vi "Find Closest Index.vi"(10 "Time":dbl, 11 "Array":dbl[][](array[numeric])) -> (3 "Index":i32)   [LabVIEW 2015]
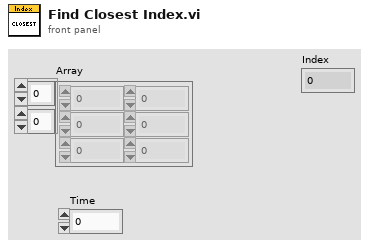
[diagram p1: front panel]
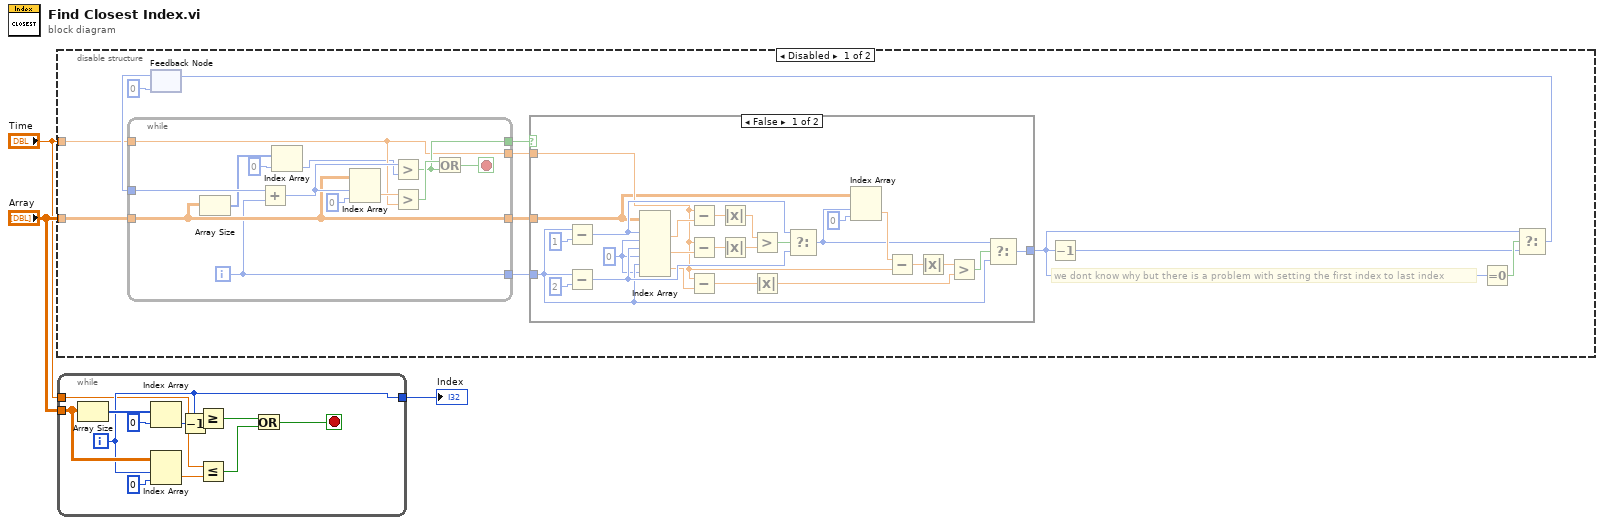
[diagram p0: block diagram]
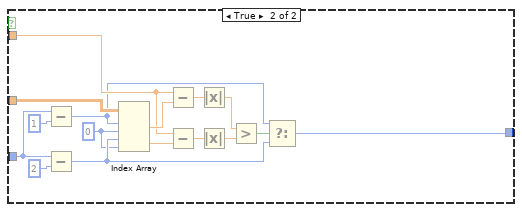
[diagram p2: hidden frame]
diagram:
  n1 = disable-structure shown="Disabled" {
    disable-tunnel: "Array" -> [w5 _]
    disable-tunnel: "Time" -> [w4 _]
    frame Disabled {
      # "we dont know why but there is a problem with setting the first index to last index"
      n2 = feedback #1(0) -> (w15:i32)
      n3 = while {
        tunnel: w5 -> [w63]
        tunnel: w15 -> [w69]
        tunnel: w4 -> [w61]
        tunnel: [w64] -> w14
        tunnel: [w63] -> w13
        tunnel: [w62] -> w12
        tunnel: [w61] -> w11
        i -> [w62]
        stop <- w65 stop-if-true
        n4 = Array Size(array=w63) -> (size(s)=w59:i32[])
        n5 = Add(x=w69, y=w62) -> (x+y=w67:i32)
        n6 = Index Array(array=w59, index=0) -> (element=w57:i32)
        n7 = Index Array(array=w63, index (row)=w67, index (col)=0 ("disabled index (col)")) -> (element=w68:dbl)
        n8 = Greater?(x=w67, y=w57) -> (0:w64:bool)
        n9 = Greater?(x=w68, y=w61) -> (0:w66:bool)
        n10 = Or(x=w66, y=w64) -> (x .or. y?=w65:bool)
      }
      n11 = case shown="False" w14 {
        tunnel: w13 -> [w23 w56]
        tunnel: w12 -> [w19 w55]
        tunnel: w11 -> [w26 w49]
        tunnel: [w18 w42] -> w6
        frame False {
          w17 = 0 ("disabled index (col)")
          n12 = Subtract(x=w19, y=1) -> (x-y=w35:i32)
          n13 = Subtract(x=w19, y=2) -> (x-y=w34:i32)
          n14 = Index Array(array=w23, index (row) #1=w35, index (col) #1=w17, index (row) #2=w34, index (col) #2=w17, index (row) #3=w19, index (col) #3=w17) -> (element #1=w33:dbl, element #2=w32:dbl, element #3=w28:dbl)
          n15 = Subtract(x=w26, y=w33) -> (x-y=w37:dbl)
          n16 = Subtract(x=w26, y=w32) -> (x-y=w38:dbl)
          n17 = Subtract(x=w26, y=w28) -> (x-y=w29:dbl)
          n18 = Absolute Value(x=w37) -> (abs(x)=w31:dbl)
          n19 = Absolute Value(x=w38) -> (abs(x)=w30:dbl)
          n20 = Greater?(x=w31, y=w30) -> (0:w36:bool)
          n21 = Absolute Value(x=w29) -> (abs(x)=w24:dbl)
          n22 = Select(t=w35, s=w36, f=w34) -> (s? t:f=w20:i32)
          n23 = Index Array(array=w23, index (row)=w20, index (col)=0 ("disabled index (col)")) -> (element=w22:dbl)
          n24 = Subtract(x=w22, y=w26) -> (x-y=w27:dbl)
          n25 = Absolute Value(x=w27) -> (abs(x)=w25:dbl)
          n26 = Greater?(x=w25, y=w24) -> (0:w21:bool)
          n27 = Select(t=w20, s=w21, f=w19) -> (s? t:f=w18:i32)
        }
        frame True {
          w41 = 0 ("disabled index (col)")
          n28 = Subtract(x=w55, y=1) -> (x-y=w44:i32)
          n29 = Subtract(x=w55, y=2) -> (x-y=w43:i32)
          n30 = Index Array(array=w56, index (row) #1=w44, index (col) #1=w41, index (row) #2=w43, index (col) #2=w41) -> (element #1=w50:dbl, element #2=w48:dbl)
          n31 = Subtract(x=w49, y=w50) -> (x-y=w52:dbl)
          n32 = Subtract(x=w49, y=w48) -> (x-y=w51:dbl)
          n33 = Absolute Value(x=w52) -> (abs(x)=w47:dbl)
          n34 = Absolute Value(x=w51) -> (abs(x)=w46:dbl)
          n35 = Greater?(x=w47, y=w46) -> (0:w45:bool)
          n36 = Select(t=w44, s=w45, f=w43) -> (s? t:f=w42:i32)
        }
      }
      n37 = Decrement(x=w6) -> (x-1=w8:i32)
      n38 = Equal To 0?(x=w6) -> (x = 0?=w9:bool)
      n39 = Select(t=w6, s=w9, f=w8) -> (s? t:f=w7:i32)
      n40 = feedback-in #1(w7) -> ()
    }
    frame Enabled {
    }
  }
  n41 = while {
    tunnel: "Array" -> [w79]
    tunnel: "Time" -> [w71]
    tunnel: [w72] -> w1
    i -> [w72]
    stop <- w76 stop-if-true
    n42 = Array Size(array=w79) -> (size(s)=w75:i32[])
    n43 = Index Array(array=w75, index=0) -> (element=w73:i32)
    n44 = Index Array(array=w79, index (row)=w72, index (col)=0 ("disabled index (col)")) -> (element=w77:dbl)
    n45 = Decrement(x=w73) -> (x-1=w70:i32)
    n46 = Greater Or Equal?(x=w72, y=w70) -> (x >= y?=w81:bool)
    n47 = Less Or Equal?(x=w71, y=w77) -> (x <= y?=w80:bool)
    n48 = Or(x=w81, y=w80) -> (x .or. y?=w76:bool)
  }
  "Index" <- w1
